vi "02.2 Tag channels.vi"() -> ()   [LabVIEW 2019]
uses:
  <extravilib>/ChannelInstances/Tag-bool/Instantiate.vi
  <extravilib>/ChannelInstances/Tag-bool/EndpointRead.vi
  <extravilib>/ChannelInstances/Tag-bool/Endpoint.vi
  <extravilib>/ChannelInstances/Tag-i32/Instantiate.vi
  <extravilib>/ChannelInstances/Tag-i32/EndpointRead.vi
  <extravilib>/ChannelInstances/Tag-i32/Endpoint.vi
  <extravilib>/ChannelInstances/Tag-i32.lvlib
  <extravilib>/ChannelInstances/Tag-bool.lvlib
panel:
  in  "Stop 2":bool
  out "Chart A 2":dbl(graph)
  out "Chart B 2":dbl(graph)
  out "Chart B":i32(graph)
  in  "Stop":bool
  out "Chart A":i32(graph)
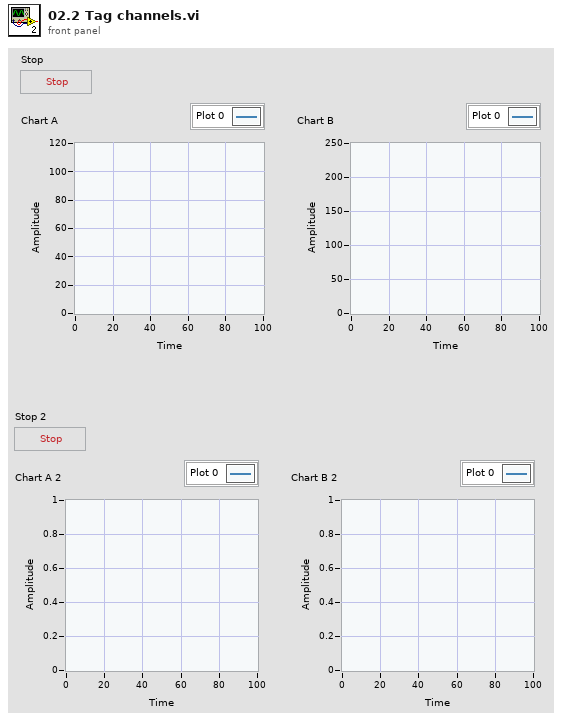
[diagram p1: front panel]
types:
  T1 = typedef "Tag-bool.lvlib/))Channel.ctl" = refnum<queue>
  T2 = typedef "Tag-i32.lvlib/))Channel.ctl" = refnum<queue>
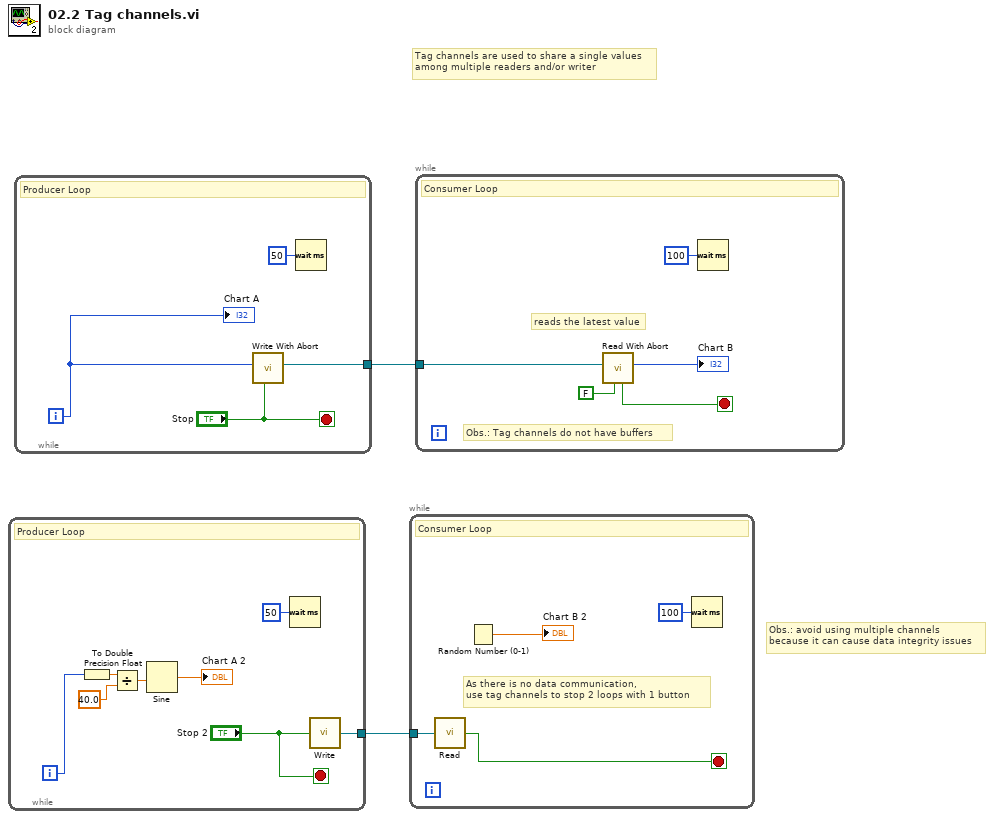
[diagram p0: block diagram]
diagram:
  # "Obs.: avoid using multiple channels\nbecause it can cause data integrity issues"
  # "Tag channels are used to share a single values\namong multiple readers and/or writer"
  n1 = while {
    tunnel: [w3] -> w1
    i -> [w6]
    stop <- "Stop 2" stop-if-true
    # "Producer Loop"
    n2 = To Double Precision Float(number=w6) -> (double precision float=w7:dbl)
    n3 = Divide(x=w7, y=40.0) -> (x/y=w8:dbl)
    n4 = Sine(x=w8) -> (sin(x)=→"Chart A 2":dbl)
    n5 = Wait (ms)(milliseconds to wait=u32 50) -> ()  [unwired: 1 out]
    n6 = call <extravilib>:"Write.vi"("element"="Stop 2") -> ("channel"=w3:T1)  [unwired: 1 out]
  }
  n7 = while {
    tunnel: [w13] -> w2
    i -> [w12]
    stop <- "Stop" stop-if-true
    # "Producer Loop"
    n8 = call <extravilib>:"Write With Abort.vi"("abort"="Stop", "element"=w12) -> ("channel"=w13:T2)  [unwired: 7 in, 2 out]
    n9 = Wait (ms)(milliseconds to wait=u32 50) -> ()  [unwired: 1 out]
    "Chart A" <- w12
  }
  n10 = while {
    tunnel: w1 -> [w16]
    stop <- w15 stop-if-true
    # "As there is no data communication,\nuse tag channels to stop 2 loops with 1 button"
    # "Consumer Loop"
    n11 = call <extravilib>:"Read.vi"("channel"=w16) -> ("element"=w15:bool)  [unwired: 1 in, 1 out]
    n12 = Random Number (0-1)() -> (number: 0 to 1=→"Chart B 2":dbl)
    n13 = Wait (ms)(milliseconds to wait=u32 100) -> ()  [unwired: 1 out]
  }
  n14 = while {
    tunnel: w2 -> [w22]
    stop <- w20 stop-if-true
    # "Obs.: Tag channels do not have buffers"
    # "reads the latest value"
    # "Consumer Loop"
    n15 = call <extravilib>:"Read With Abort.vi"("abort"=FALSE, "channel"=w22) -> ("element"=→"Chart B":i32, "aborted?"=w20:bool)  [unwired: 7 in, 1 out]
    n16 = Wait (ms)(milliseconds to wait=u32 100) -> ()  [unwired: 1 out]
  }
